vi "Write Public Events.vi"(8 "error in (no error)":errorcluster, 10 "Public Events":T1, 11 "Test Assert Factory in":refnum<class "Test Assert Factory.lvclass">) -> (0 "error out":errorcluster, 3 "Test Assert Factory out":refnum<class "Test Assert Factory.lvclass">)   [LabVIEW 2013, in "Caraya.lvlib" / "Test Assert Factory.lvclass"]
uses:
  Test Assert Factory.lvclass
  Test Result/Test Events -- cluster.ctl
  Test Assert Factory.lvclass/Test Assert Factory.ctl
  Test Result/Test Result.lvclass
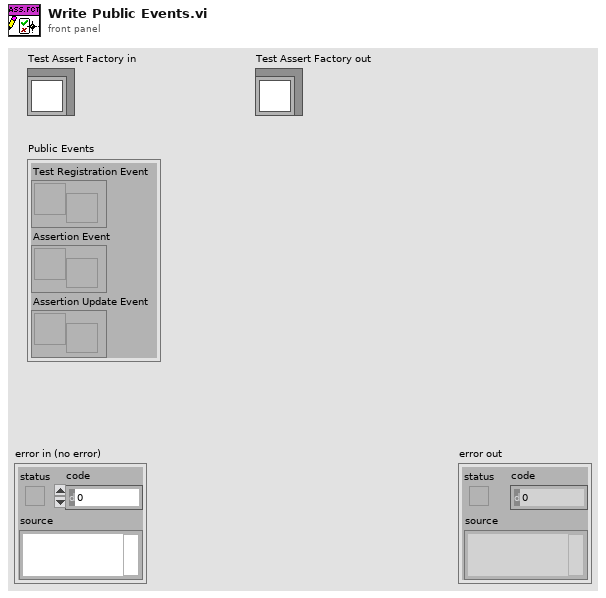
[diagram p1: front panel]
types:
  T1 = typedef "Caraya.lvlib/Test Result.lvclass/Test Events -- cluster.ctl" = cluster{"Test Registration Event":refnum<user-event>, "Assertion Event":refnum<user-event>, "Assertion Update Event":refnum<user-event>}
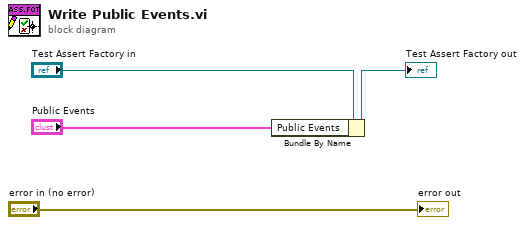
[diagram p0: block diagram]
diagram:
  n1 = Bundle By Name(cluster="Test Assert Factory in", "Public Events"="Public Events") -> (→"Test Assert Factory out":refnum<class "Test Assert Factory.lvclass">)
  "error out" <- "error in (no error)"
